vi "Begin Auton.vi"   [LabVIEW 2012]
uses:
  <vilib>/Rock Robotics/SystemInterfaces/DIO/FPGA_DIOChannel.ctl
  <vilib>/Rock Robotics/SystemInterfaces/Typedef/FPGA_TypedefDigitalModule.ctl
types:
  T1 = typedef "FPGA_DIOChannel.ctl" = enum8{"DIO 1", "DIO 2", "DIO 3", "DIO 4", "DIO 5", "DIO 6", "DIO 7", "DIO 8", "DIO 9", "DIO 10", "DIO 11", "DIO 12", "DIO 13", "DIO 14", "Invalid"}
  T2 = typedef "FPGA_TypedefDigitalModule.ctl" = enum16{"Digital Module 1", "Digital Module 2"}
  T3 = typedef "WPI_DigitalInputDevRef.ctl" = cluster{"DevStatus":errorcluster, "DIO Channel":T1, "Digital Module":T2}
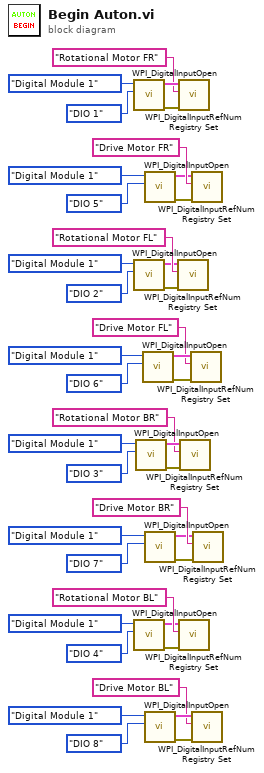
[diagram p0: block diagram]
diagram:
  n1 = call <vilib>:"WPI_DigitalInputOpen.vi"("DIO Channel"=FPGA_DIOChannel."DIO 1", "Digital Module (Module 1)"=FPGA_TypedefDigitalModule."Digital Module 1") -> ("error out"=w39:errorcluster, "DigitalInputDevRef"=w40:T3)  [unwired: 8 in]
  n2 = call <vilib>:"WPI_DigitalInputOpen.vi"("DIO Channel"=FPGA_DIOChannel."DIO 2", "Digital Module (Module 1)"=FPGA_TypedefDigitalModule."Digital Module 1") -> ("error out"=w32:errorcluster, "DigitalInputDevRef"=w31:T3)  [unwired: 8 in]
  n3 = call <vilib>:"WPI_DigitalInputOpen.vi"("DIO Channel"=FPGA_DIOChannel."DIO 4", "Digital Module (Module 1)"=FPGA_TypedefDigitalModule."Digital Module 1") -> ("error out"=w22:errorcluster, "DigitalInputDevRef"=w21:T3)  [unwired: 8 in]
  n4 = call <vilib>:"WPI_DigitalInputOpen.vi"("DIO Channel"=FPGA_DIOChannel."DIO 3", "Digital Module (Module 1)"=FPGA_TypedefDigitalModule."Digital Module 1") -> ("error out"=w29:errorcluster, "DigitalInputDevRef"=w30:T3)  [unwired: 8 in]
  n5 = call <vilib>:"WPI_DigitalInputOpen.vi"("DIO Channel"=FPGA_DIOChannel."DIO 6", "Digital Module (Module 1)"=FPGA_TypedefDigitalModule."Digital Module 1") -> ("error out"=w9:errorcluster, "DigitalInputDevRef"=w10:T3)  [unwired: 8 in]
  n6 = call <vilib>:"WPI_DigitalInputOpen.vi"("DIO Channel"=FPGA_DIOChannel."DIO 5", "Digital Module (Module 1)"=FPGA_TypedefDigitalModule."Digital Module 1") -> ("error out"=w2:errorcluster, "DigitalInputDevRef"=w1:T3)  [unwired: 8 in]
  n7 = call <vilib>:"WPI_DigitalInputOpen.vi"("DIO Channel"=FPGA_DIOChannel."DIO 7", "Digital Module (Module 1)"=FPGA_TypedefDigitalModule."Digital Module 1") -> ("error out"=w12:errorcluster, "DigitalInputDevRef"=w11:T3)  [unwired: 8 in]
  n8 = call <vilib>:"WPI_DigitalInputOpen.vi"("DIO Channel"=FPGA_DIOChannel."DIO 8", "Digital Module (Module 1)"=FPGA_TypedefDigitalModule."Digital Module 1") -> ("error out"=w19:errorcluster, "DigitalInputDevRef"=w20:T3)  [unwired: 8 in]
  n9 = call <vilib>:"WPI_DigitalInputRefNum Registry Set.vi"("error in (no error)"=w32, "refnum name"="Rotational Motor FL", "DigitalInputDevRef"=w31) -> ()  [unwired: 7 in, 2 out]
  n10 = call <vilib>:"WPI_DigitalInputRefNum Registry Set.vi"("error in (no error)"=w39, "refnum name"="Rotational Motor FR", "DigitalInputDevRef"=w40) -> ()  [unwired: 7 in, 2 out]
  n11 = call <vilib>:"WPI_DigitalInputRefNum Registry Set.vi"("error in (no error)"=w22, "refnum name"="Rotational Motor BL", "DigitalInputDevRef"=w21) -> ()  [unwired: 7 in, 2 out]
  n12 = call <vilib>:"WPI_DigitalInputRefNum Registry Set.vi"("error in (no error)"=w29, "refnum name"="Rotational Motor BR", "DigitalInputDevRef"=w30) -> ()  [unwired: 7 in, 2 out]
  n13 = call <vilib>:"WPI_DigitalInputRefNum Registry Set.vi"("error in (no error)"=w9, "refnum name"="Drive Motor FL", "DigitalInputDevRef"=w10) -> ()  [unwired: 7 in, 2 out]
  n14 = call <vilib>:"WPI_DigitalInputRefNum Registry Set.vi"("error in (no error)"=w2, "refnum name"="Drive Motor FR", "DigitalInputDevRef"=w1) -> ()  [unwired: 7 in, 2 out]
  n15 = call <vilib>:"WPI_DigitalInputRefNum Registry Set.vi"("error in (no error)"=w19, "refnum name"="Drive Motor BL", "DigitalInputDevRef"=w20) -> ()  [unwired: 7 in, 2 out]
  n16 = call <vilib>:"WPI_DigitalInputRefNum Registry Set.vi"("error in (no error)"=w12, "refnum name"="Drive Motor BR", "DigitalInputDevRef"=w11) -> ()  [unwired: 7 in, 2 out]
